vi "GA_Create Population.vi"(5 "ClassifierClass.lvclass":refnum<class "ClassifierClass.lvclass">, 7 "Fitness Function":T2, 8 "Phenotype size":i32, 9 "Population size":i32) -> (3 "Population out":T1)   [LabVIEW 2016, in "GA.lvlib"]
doc: "Randomizes population and calculate fitnesses"
uses:
  GA.lvlib
  GA_tFitness Function.ctl
  4. Accuracy Assessment for EEG Classification/_vlib/ClassifierClass.lvclass
  GA_tPopulation.ctl
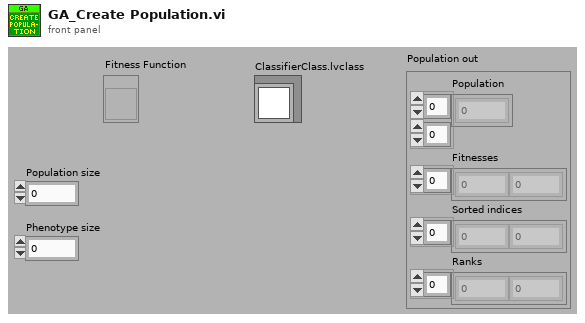
[diagram p1: front panel]
types:
  T1 = typedef "GA.lvlib/GA_tPopulation.ctl" = cluster{"Population":i8[][], "Fitnesses":dbl[], "Sorted indices":i32[], "Ranks":i32[]}
  T2 = typedef "GA.lvlib/GA_tFitness Function.ctl" = refnum<vi>
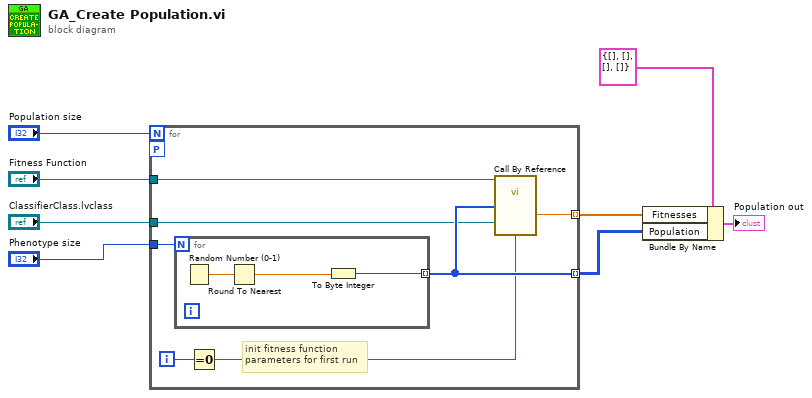
[diagram p0: block diagram]
diagram:
  n1 = for {
    N: "Population size" -> [_]
    tunnel: "Phenotype size" -> [w15]
    tunnel: "Fitness Function" -> [w11]
    tunnel: [w13] -> w4 mode=indexing
    tunnel: [w14] -> w3 mode=indexing
    tunnel: "ClassifierClass.lvclass" -> [w12]
    workers-P: _ -> [_]
    i -> [w10]
    # "init fitness function\nparameters for first run"
    n2 = for {
      N: w15 -> [_]
      tunnel: [w16] -> w14 mode=indexing
      n3 = Random Number (0-1)() -> (number: 0 to 1=w18:dbl)
      n4 = Round To Nearest(number=w18) -> (nearest integer value=w17:dbl)
      n5 = To Byte Integer(number=w17) -> (8bit integer=w16:i8)
    }
    n6 = Equal To 0?(x=w10) -> (x = 0?=w9:bool)
    n7 = call-by-ref "?"(reference=w11, "Init? (F)"=w9, "ClassifierClass.lvclass"=w12, "Phenotype"=w14) -> ("Fitness"=w13:dbl)  [unwired: 1 in, 2 out]
  }
  n8 = Bundle By Name(cluster=T1 {"Population"=[], "Fitnesses"=[], "Sorted indices"=[], "Ranks"=[]} ("Population out"), "Fitnesses"=w4, "Population"=w3) -> (→"Population out":T1)
